vi "Start Server.vi"(8 "error in (no error)":errorcluster, 11 "gRPC Server in":refnum<class "Query Server.lvclass">) -> (0 "error out":errorcluster, 3 "gRPC Server out":refnum<class "Query Server.lvclass">)   [LabVIEW 2016, in "Query Server.lvlib" / "Query Server.lvclass"]
uses:
  Query Server.lvclass
  gRPC lvSupport/gprc-lvsupport.lvlib
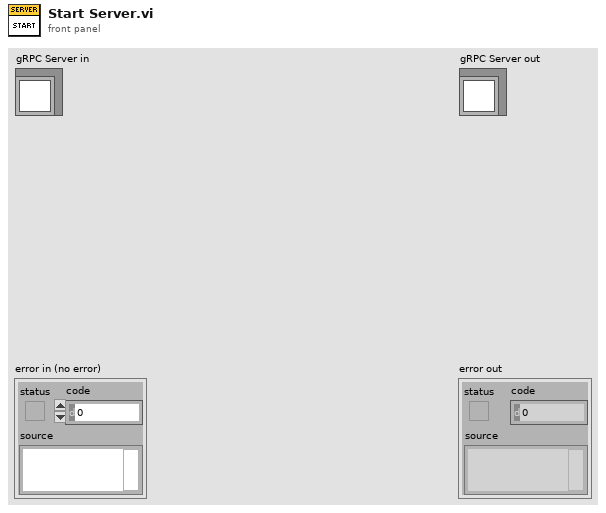
[diagram p1: front panel]
types:
  T1 = typedef "Query Server.lvlib/gprc-lvsupport.lvlib/grpcId.ctl" = u64
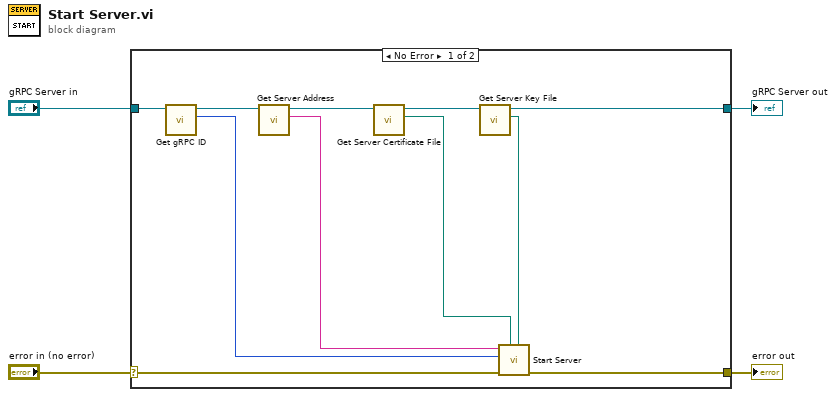
[diagram p0: block diagram]
diagram:
  n1 = case shown="No Error" "error in (no error)" {
    selector: "error in (no error)" -> [w15 w17]
    tunnel: [w5 w17] -> w3
    tunnel: [w6 w16] -> w1
    tunnel: "gRPC Server in" -> [w13 w16]
    frame No Error {
      n2 = call "Get gRPC ID.vi"("OOP Server in"=w13) -> ("gRPC ID"=w11:T1, "OOP Server out"=w12:refnum<class "Query Server.lvclass">)  [unwired: 9 in]
      n3 = call "Get Server Address.vi"("OOP Server in"=w12) -> ("Server Address"=w14:string, "OOP Server out"=w10:refnum<class "Query Server.lvclass">)  [unwired: 9 in]
      n4 = call "Get Server Certificate File.vi"("OOP Server in"=w10) -> ("Server Certificate File (.crt)"=w9:path, "OOP Server out"=w8:refnum<class "Query Server.lvclass">)  [unwired: 9 in]
      n5 = call "Get Server Key File.vi"("OOP Server in"=w8) -> ("Server Key File (.key)"=w7:path, "OOP Server out"=w6:refnum<class "Query Server.lvclass">)  [unwired: 9 in]
      n6 = call "Start Server.vi"("Server Key File (.key)"=w7, "Server Certificate File (.crt)"=w9, "error in (no error)"=w15, "gRPCid"=w11, "Server Address"=w14) -> ("error out"=w5:errorcluster)  [unwired: 6 in]
    }
    frame Error {
    }
  }
  "error out" <- w3
  "gRPC Server out" <- w1
